vi "waveformparamsv2.vi"(0 "command":string="clear", 1 "Params in":T5, 2 "add AO":T4(array[cluster]), 3 "add DO":T3(array[cluster]), 4 "index":i32) -> (5 "Params out":T5, 6 "last AO":T2, 7 "last DO":T1)   [LabVIEW 2015]
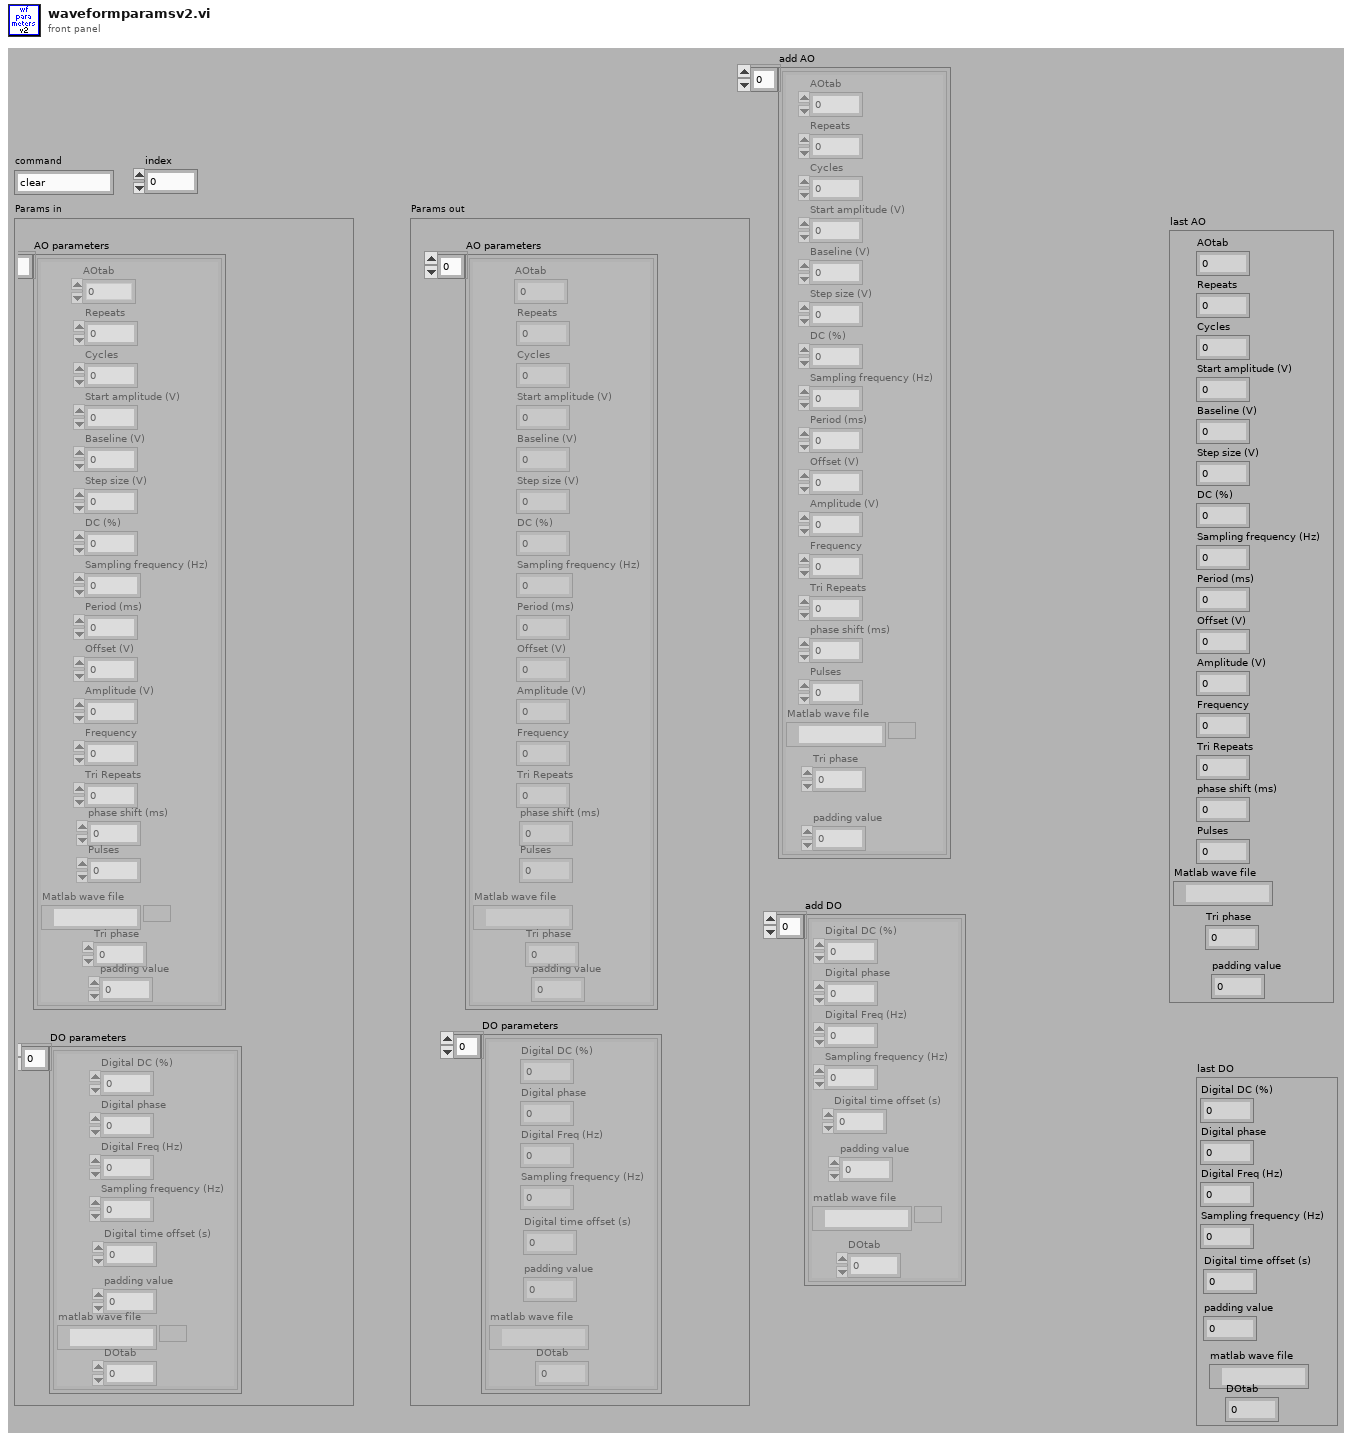
[diagram p1: front panel]
types:
  T1 = cluster{"Digital DC (%)":dbl, "Digital phase":dbl, "Digital Freq (Hz)":dbl, "Sampling frequency (Hz)":dbl, "Digital time offset (s) ":dbl, "padding value":dbl, "matlab wave file":path, "DOtab":dbl}
  T2 = cluster{"AOtab":dbl, "Repeats":dbl, "Cycles":dbl, "Start amplitude (V)":dbl, "Baseline (V)":dbl, "Step size (V)":dbl, "DC (%)":dbl, "Sampling frequency (Hz)":dbl, "Period (ms)":dbl, "Offset (V)":dbl, "Amplitude (V)":dbl, "Frequency":dbl, "Tri Repeats":dbl, "phase shift (ms)":dbl, "Pulses":dbl, "Matlab wave file":path, "Tri phase":dbl, "padding value":dbl}
  T3 = cluster{"Digital DC (%)":dbl, "Digital phase":dbl, "Digital Freq (Hz)":dbl, "Sampling frequency (Hz)":dbl, "Digital time offset (s) ":dbl, "padding value":dbl, "matlab wave file":path, "DOtab":dbl}[]
  T4 = cluster{"AOtab":dbl, "Repeats":dbl, "Cycles":dbl, "Start amplitude (V)":dbl, "Baseline (V)":dbl, "Step size (V)":dbl, "DC (%)":dbl, "Sampling frequency (Hz)":dbl, "Period (ms)":dbl, "Offset (V)":dbl, "Amplitude (V)":dbl, "Frequency":dbl, "Tri Repeats":dbl, "phase shift (ms)":dbl, "Pulses":dbl, "Matlab wave file":path, "Tri phase":dbl, "padding value":dbl}[]
  T5 = cluster{"AO parameters":cluster{"AOtab":dbl, "Repeats":dbl, "Cycles":dbl, "Start amplitude (V)":dbl, "Baseline (V)":dbl, "Step size (V)":dbl, "DC (%)":dbl, "Sampling frequency (Hz)":dbl, "Period (ms)":dbl, "Offset (V)":dbl, "Amplitude (V)":dbl, "Frequency":dbl, "Tri Repeats":dbl, "phase shift (ms)":dbl, "Pulses":dbl, "Matlab wave file":path, "Tri phase":dbl, "padding value":dbl}[], "DO parameters":cluster{"Digital DC (%)":dbl, "Digital phase":dbl, "Digital Freq (Hz)":dbl, "Sampling frequency (Hz)":dbl, "Digital time offset (s) ":dbl, "padding value":dbl, "matlab wave file":path, "DOtab":dbl}[]}
  T6 = cluster{"AOtab":dbl, "Repeats":dbl, "Cycles":dbl, "Start amplitude (V)":dbl, "Baseline (V)":dbl, "Step size (V)":dbl, "DC (%)":dbl, "Sampling frequency (Hz)":dbl, "Period (ms)":dbl, "Offset (V)":dbl, "Amplitude (V)":dbl, "Frequency":dbl, "Tri Repeats":dbl, "Cycle length (s)":dbl, "Pulses":dbl, "Matlab wave file":path, "Tri phase":dbl, "padding value":dbl}[]
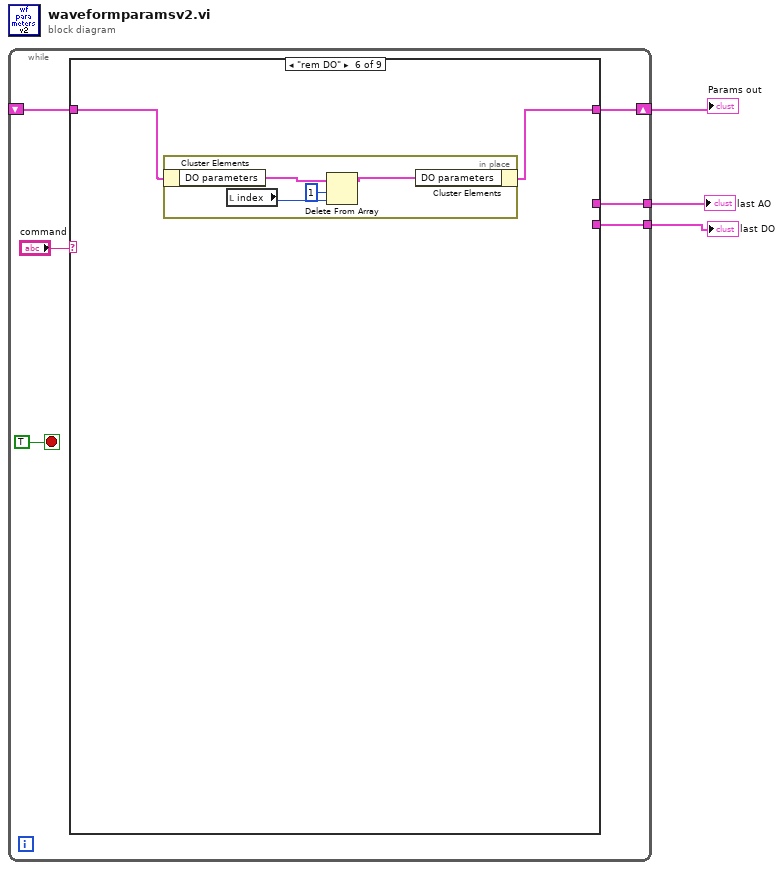
[diagram p0: block diagram]
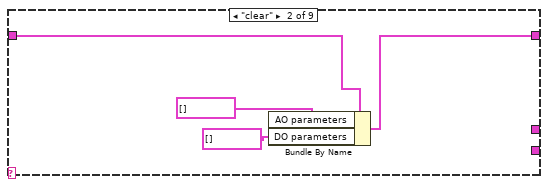
[diagram p3: hidden frame]
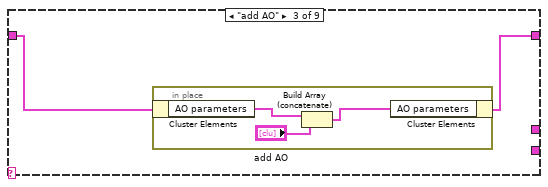
[diagram p4: hidden frame]
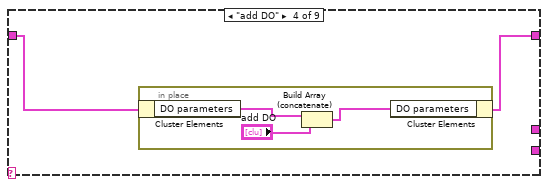
[diagram p5: hidden frame]
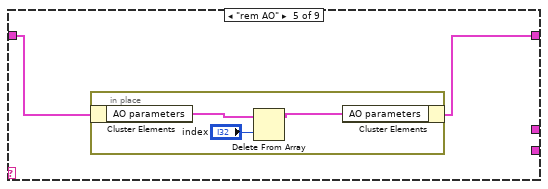
[diagram p6: hidden frame]
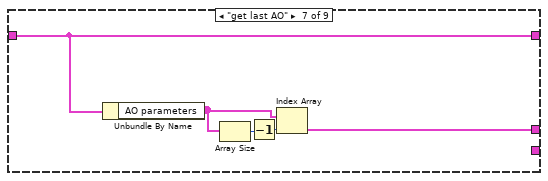
[diagram p7: hidden frame]
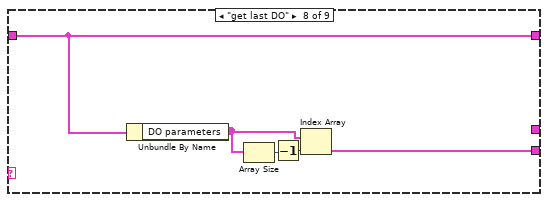
[diagram p8: hidden frame]
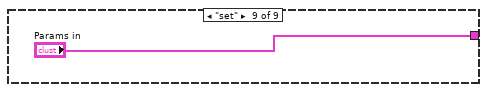
[diagram p9: hidden frame]
diagram:
  n1 = while {
    shift-right: [w7] -> w3
    shift-left: _ -> [w6]
    tunnel: [w5] -> w2
    tunnel: [w4] -> w1
    stop <- TRUE stop-if-true
    n2 = case shown="\"rem DO\"" "command" {
      tunnel: [w10 w13 w15 w20 w25 w30 w38 w42 "Params in"] -> w7
      tunnel: w6 -> [w10 w14 w16 w21 w26 w31 w38 w42 _]
      tunnel: [_ _ _ _ _ _ w36 _ _] -> w5
      tunnel: [_ _ _ _ _ _ _ w41 _] -> w4
      frame "get", Default {
      }
      frame "clear" {
        n3 = Bundle By Name(cluster=w14, "AO parameters"=T6 [], "DO parameters"=T3 []) -> (w13:T5)
      }
      frame "add AO" {
        n4 = in-place {
          n5 = in-place-cluster #1(w16) -> ("AO parameters"=w19:T4)
          n6 = Build Array (concatenate)(w19, "add AO") -> (w18:T4)
          n7 = in-place-cluster #1("AO parameters"=w18) -> (w15:T5)
        }
      }
      frame "add DO" {
        n8 = in-place {
          n9 = in-place-cluster #2(w21) -> ("DO parameters"=w24:T3)
          n10 = Build Array (concatenate)(w24, "add DO") -> (w23:T3)
          n11 = in-place-cluster #2("DO parameters"=w23) -> (w20:T5)
        }
      }
      frame "rem AO" {
        n12 = in-place {
          n13 = in-place-cluster #3(w26) -> ("AO parameters"=w29:T4)
          n14 = Delete From Array(array=w29, index="index") -> (array with subset deleted=w28:T4)  [unwired: 1 in, 1 out]
          n15 = in-place-cluster #3("AO parameters"=w28) -> (w25:T5)
        }
      }
      frame "rem DO" {
        n16 = in-place {
          n17 = in-place-cluster #4(w31) -> ("DO parameters"=w35:T3)
          n18 = local read "index"() -> (w33:i32)
          n19 = Delete From Array(array=w35, length=1, index=w33) -> (array with subset deleted=w34:T3)  [unwired: 1 out]
          n20 = in-place-cluster #4("DO parameters"=w34) -> (w30:T5)
        }
      }
      frame "get last AO" {
        n21 = Unbundle By Name(w38) -> ("AO parameters"=w39:T4)
        n22 = Array Size(array=w39) -> (size(s)=w40:i32)
        n23 = Decrement(x=w40) -> (x-1=w37:i32)
        n24 = Index Array(array=w39, index=w37) -> (element=w36:T2)
      }
      frame "get last DO" {
        n25 = Unbundle By Name(w42) -> ("DO parameters"=w44:T3)
        n26 = Array Size(array=w44) -> (size(s)=w45:i32)
        n27 = Decrement(x=w45) -> (x-1=w43:i32)
        n28 = Index Array(array=w44, index=w43) -> (element=w41:T1)
      }
      frame "set" {
      }
    }
  }
  "Params out" <- w3
  "last AO" <- w2
  "last DO" <- w1
